vi "StartMeasure.vi"(1 "error in (no error)":errorcluster) -> (0 "error IO":errorcluster caption="error out")   [LabVIEW 2018]
uses:
  globalMessage.vi
  Reslut.vi
panel:
  out "偏振度":string
  out "偏振方向":string
  out "功率输出":string
  out "能量输出":string
  out "当前信息":string
  out "完成？":bool
  out "提示":string
  out "激光器状态":i32[](listbox)
  # "能量"
  # "功率"
  # "偏振方向"
  # "偏振度"
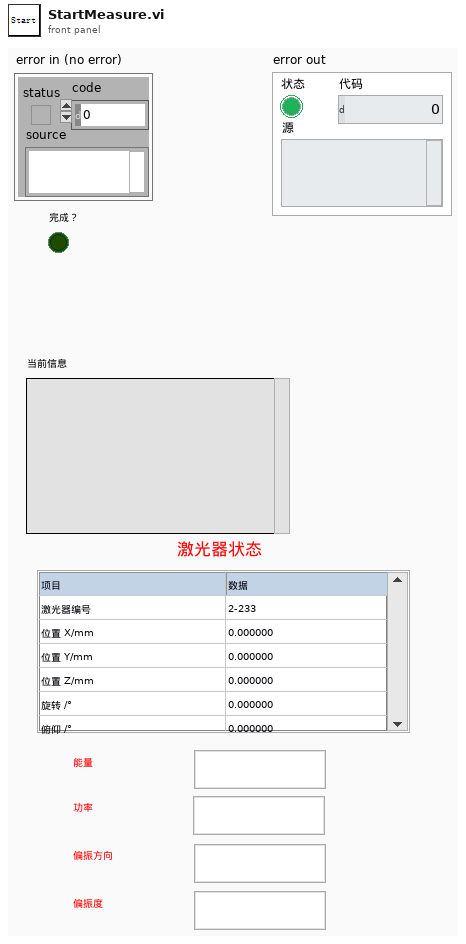
[diagram p1: front panel]
types:
  T1 = cluster{"Selected Index []":i32[], "Selected Items":string[]}
  T2 = enum16{"功率测量", "能量测量", "光谱测量", "时间波形", "偏振测量", "近远场"}
  T3 = cluster{"激光器型号":string, "X":dbl, "Y":dbl, "Z":dbl, "Rotate":dbl, "Pitching":dbl}
  T4 = cluster{"能量计结果":string, "功率计结果":string, " 偏振方向":string, "偏振度":string}
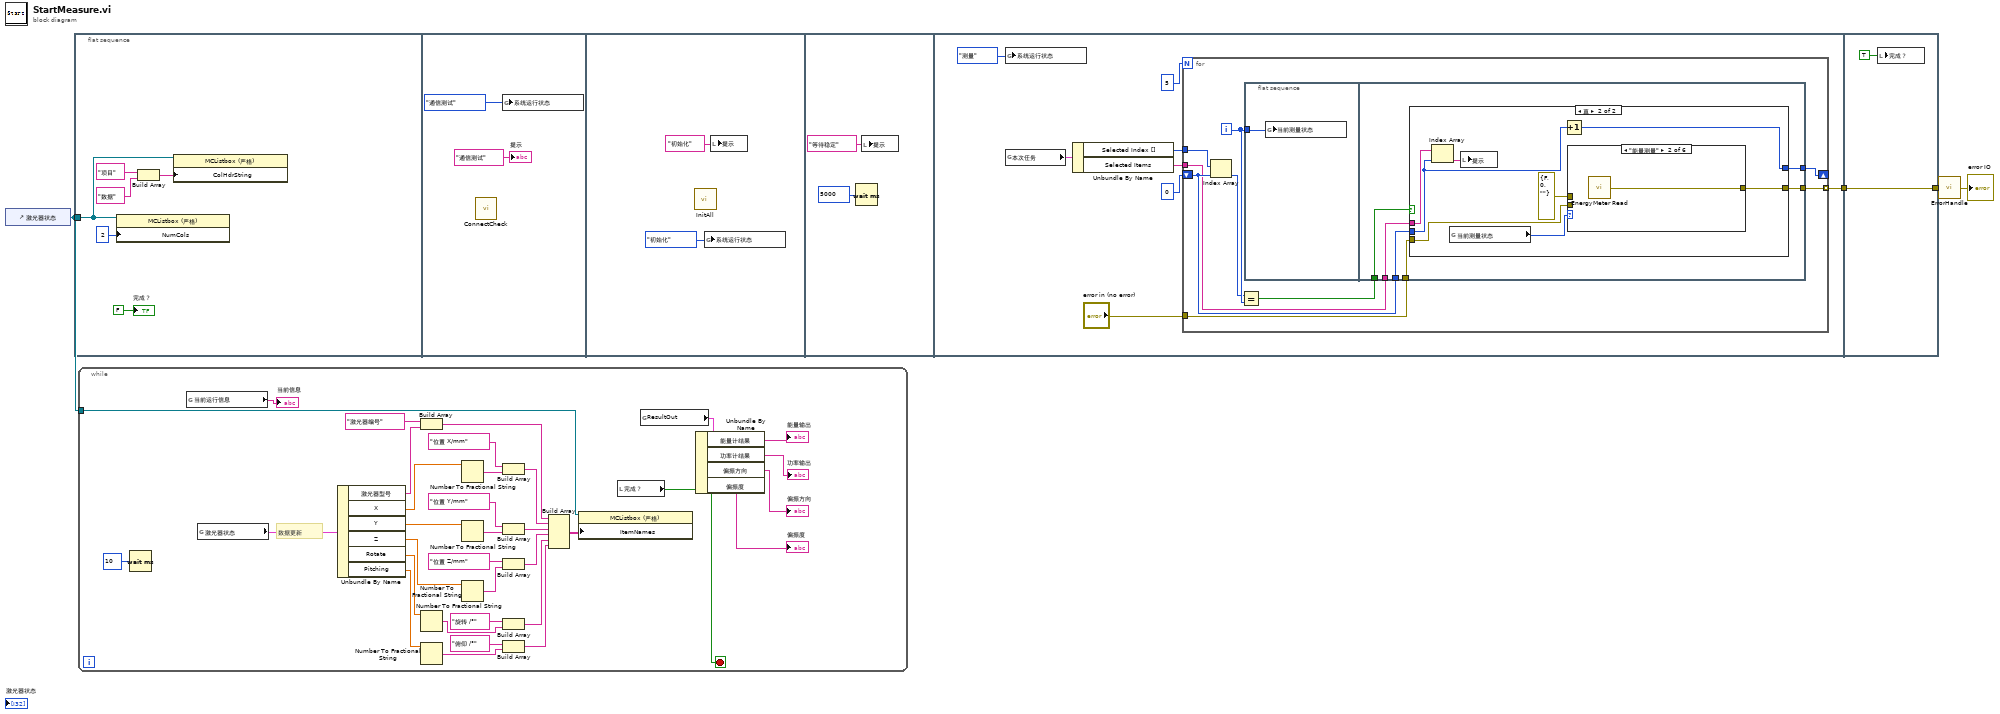
[diagram p0: block diagram]
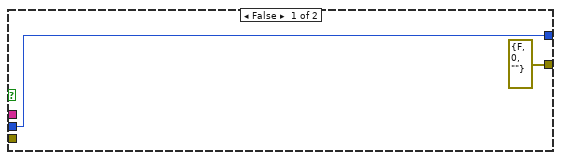
[diagram p2: hidden frame]
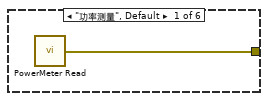
[diagram p3: hidden frame]
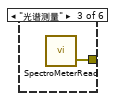
[diagram p4: hidden frame]
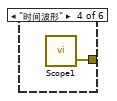
[diagram p5: hidden frame]
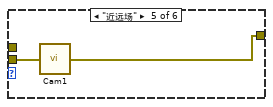
[diagram p6: hidden frame]
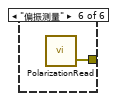
[diagram p7: hidden frame]
diagram:
  n1 = control-ref of="激光器状态"() -> (w1:refnum<vi>)
  n2 = flat-sequence {
    tunnel: w1 -> [w5]
    tunnel: [w20] -> w2
    tunnel: [w59] -> w4
    tunnel: w2 -> [w59]
    frame #0 {
      n3 = property on="属性节点" class="MCListbox (严格)"(reference=w5, "NumCols"=u32 2 ("列数")) -> ()  [unwired: 1 in, 2 out]
      n4 = Build Array("项目", "数据") -> (w9:string[])
      n5 = property on="属性节点" class="MCListbox (严格)"(reference=w5, "ColHdrString"=w9) -> ()  [unwired: 1 in, 2 out]
      "完成？" <- FALSE
    }
    frame #1 {
      n6 = call "ConnectCheck.vi"() -> ()  [unwired: 12 in]
      n7 = global write "参数.vi" "系统运行状态"(enum16{"通信测试", "初始化", "测量", "写入"}."通信测试" ("系统运行状态")) -> ()
      "提示" <- "通信测试" ("提示")
    }
    frame #2 {
      n8 = call "InitAll.vi"() -> ()  [unwired: 3 in, 1 out]
      n9 = global write "参数.vi" "系统运行状态"(enum16{"通信测试", "初始化", "测量", "写入"}."初始化" ("系统运行状态")) -> ()
      n10 = local write "提示"("初始化" ("提示")) -> ()
    }
    frame #3 {
      n11 = Wait (ms)(milliseconds to wait=u32 5000 ("等待时间（毫秒）")) -> ()  [unwired: 1 out]
      n12 = local write "提示"("等待稳定" ("提示")) -> ()
    }
    frame #4 {
      n13 = global write "参数.vi" "系统运行状态"(enum16{"通信测试", "初始化", "测量", "写入"}."测量" ("系统运行状态")) -> ()
      n14 = global read "参数.vi" "本次任务"() -> (w22:T1)
      n15 = Unbundle By Name(w22) -> ("Selected Index []"=w21:i32[], "Selected Items"=w18:string[])
      n16 = for {
        N: 5 -> [_]
        tunnel: w21 -> [w33]
        shift-right: [w29] -> _
        shift-left: 0 -> [w27]
        tunnel: [w28] -> w20 mode=indexing
        tunnel: "error in (no error)" -> [w26]
        tunnel: w18 -> [w25]
        i -> [w32]
        n17 = Index Array(array=w33, index=w27) -> (element=w30:i32)
        n18 = Equal?(x=w30, y=w32) -> (x = y?=w31:bool)
        n19 = flat-sequence {
          tunnel: w32 -> [w34]
          tunnel: w31 -> [w40]
          tunnel: w27 -> [w39]
          tunnel: [w38] -> w29
          tunnel: [w37] -> w28
          tunnel: w26 -> [w36]
          tunnel: w25 -> [w35]
          frame #0 {
            n20 = global write "参数.vi" "当前测量状态"(w34) -> ()
          }
          frame #1 {
            n21 = case shown="真" w40 {
              tunnel: w39 -> [w42 w44]
              tunnel: [w42 w50] -> w38
              tunnel: [errorcluster {"status"=FALSE, "code"=0, "source"=""} ("error out") w47] -> w37
              tunnel: w36 -> [_ w46]
              tunnel: w35 -> [_ w45]
              frame False {
              }
              frame True {
                n22 = Index Array(array=w45, index=w44) -> (element=w43:string)
                n23 = global read "参数.vi" "当前测量状态"() -> (w49:T2)
                n24 = local write "提示"(w43) -> ()
                n25 = Increment(x=w44) -> (x+1=w50:i32)
                n26 = case shown="\"能量测量\"" w49 {
                  tunnel: [w51 w52 w53 w54 w56 w57] -> w47
                  tunnel: errorcluster {"status"=FALSE, "code"=0, "source"=""} ("error out") -> [_ _ _ _ _ _]
                  tunnel: w46 -> [_ _ _ _ w55 _]
                  frame "功率测量", Default {
                    n27 = call "PowerMeter Read.vi"() -> ("错误输出"=w51:errorcluster)  [unwired: 3 in, 1 out]
                  }
                  frame "能量测量" {
                    n28 = call "EnergyMeter Read.vi"() -> ("错误输出"=w52:errorcluster)  [unwired: 3 in, 2 out]
                  }
                  frame "光谱测量" {
                    n29 = call "SpectroMeterRead.vi"() -> ("error out"=w53:errorcluster)  [unwired: 3 in]
                  }
                  frame "时间波形" {
                    n30 = call "Scope1.vi"() -> ("错误输出"=w54:errorcluster)  [unwired: 3 in]
                  }
                  frame "近远场" {
                    n31 = call "Cam1.vi"("error in (no error)"=w55) -> ("error out"=w56:errorcluster)
                  }
                  frame "偏振测量" {
                    n32 = call "PolarizationRead.vi"() -> ("error IO 2"=w57:errorcluster)  [unwired: 3 in]
                  }
                }
              }
            }
          }
        }
      }
    }
    frame #5 {
      n33 = local write "完成？"(TRUE ("完成？")) -> ()
    }
  }
  n34 = while {
    tunnel: w1 -> [w66]
    stop <- w67 stop-if-true
    # "数据更新"
    n35 = Wait (ms)(milliseconds to wait=u32 10 ("等待时间（毫秒）")) -> ()  [unwired: 1 out]
    n36 = global read "globalMessage.vi" "当前运行信息"() -> (→"当前信息":string)
    n37 = global read "参数.vi" "激光器状态"() -> (w80:T3)
    n38 = Unbundle By Name(w80) -> ("激光器型号"=w79:string, "X"=w78:dbl, "Y"=w76:dbl, "Z"=w75:dbl, "Rotate"=w74:dbl, "Pitching"=w73:dbl)
    n39 = Build Array("激光器编号", w79) -> (w87:string[])
    n40 = Number To Fractional String(number=w74) -> (F-format string=w70:string)  [unwired: 3 in]
    n41 = Number To Fractional String(number=w73) -> (F-format string=w69:string)  [unwired: 3 in]
    n42 = Number To Fractional String(number=w78) -> (F-format string=w77:string)  [unwired: 3 in]
    n43 = Number To Fractional String(number=w76) -> (F-format string=w72:string)  [unwired: 3 in]
    n44 = Number To Fractional String(number=w75) -> (F-format string=w71:string)  [unwired: 3 in]
    n45 = Build Array("位置 X/mm", w77) -> (w86:string[])
    n46 = Build Array("位置 Y/mm", w72) -> (w85:string[])
    n47 = Build Array("位置 Z/mm", w71) -> (w84:string[])
    n48 = Build Array("旋转 /°", w70) -> (w83:string[])
    n49 = Build Array("俯仰 /°", w69) -> (w82:string[])
    n50 = Build Array(w87, w86, w85, w84, w83, w82) -> (w81:string[][])
    n51 = property on="属性节点" class="MCListbox (严格)"(reference=w66, "ItemNames"=w81) -> ()  [unwired: 1 in, 2 out]
    n52 = local read "完成？"() -> (w67:bool)
    n53 = global read "Reslut.vi" "ResultOut"() -> (w64:T4)
    n54 = Unbundle By Name(w64) -> ("能量计结果"=→"能量输出":string, "功率计结果"=→"功率输出":string, "偏振方向"=→"偏振方向":string, "偏振度"=→"偏振度":string)
  }
  n55 = call "ErrorHandle.vi"("Error"=w4) -> ("error IO"=→"error IO":errorcluster)
